vi "DT3120_CheckStatus.vi"(8 "error in":errorcluster, 11 "Status":u32) -> (0 "error out":errorcluster, 3 "New Error?":bool)   [LabVIEW 2010]
uses:
  olimg32.dll
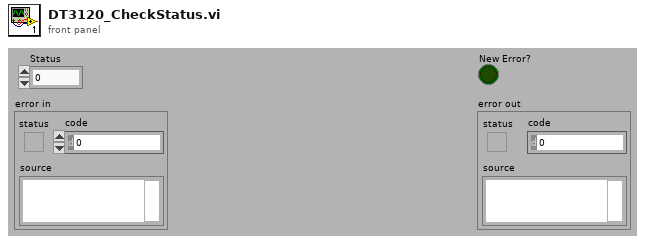
[diagram p1: front panel]
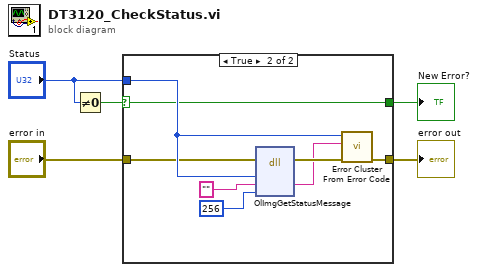
[diagram p0: block diagram]
diagram:
  n1 = Not Equal To 0?(x="Status") -> (x != 0?=w2:bool)
  n2 = case shown="True" w2 {
    selector: w2 -> [w6 w8]
    tunnel: "error in" -> [w7 w11]
    tunnel: [w7 w13] -> w4
    tunnel: "Status" -> [_ w12]
    tunnel: [w6 w8] -> w1
    frame False {
    }
    frame True {
      n3 = dll-call lib="C:/LabVIEW Programs/MT Scan PicoHarp/SubVIs/olimg32.dll" fn="OlImgGetStatusMessage"(error in=w11, "Status"=w12, "MessageBuf"="", "BufSize"=256) -> (error out=w10:errorcluster, "MessageBuf"=w9:string)  [unwired: 4 in, 2 out]
      n4 = call <vilib>:"Error Cluster From Error Code.vi"("error in (no error)"=w10, "error message (\"\")"=w9, "error code (0)"=w12) -> ("error out"=w13:errorcluster)  [unwired: 1 in, 5 out]
    }
  }
  "error out" <- w4
  "New Error?" <- w1
